vi "Generate Comments.vi"(7 "error in (no error)":errorcluster, 9 "cluster":T1) -> (0 "error out":errorcluster, 3 "Comments":string)   [LabVIEW 2016, in "Control Experiment.lvclass"]
uses:
  Control Experiment.lvclass
  Typedefs/Comments-cluster.ctl
  <userlib>/LevyLab/Krohn Hite 7008/typedefs/Gain-Enum.ctl
  <userlib>/LevyLab/Krohn Hite 7008/typedefs/Input Configuration-Enum.ctl
  <userlib>/LevyLab/Krohn Hite 7008/typedefs/Shunt-Enum.ctl
  <userlib>/LevyLab/Krohn Hite 7008/KH7008.lvclass
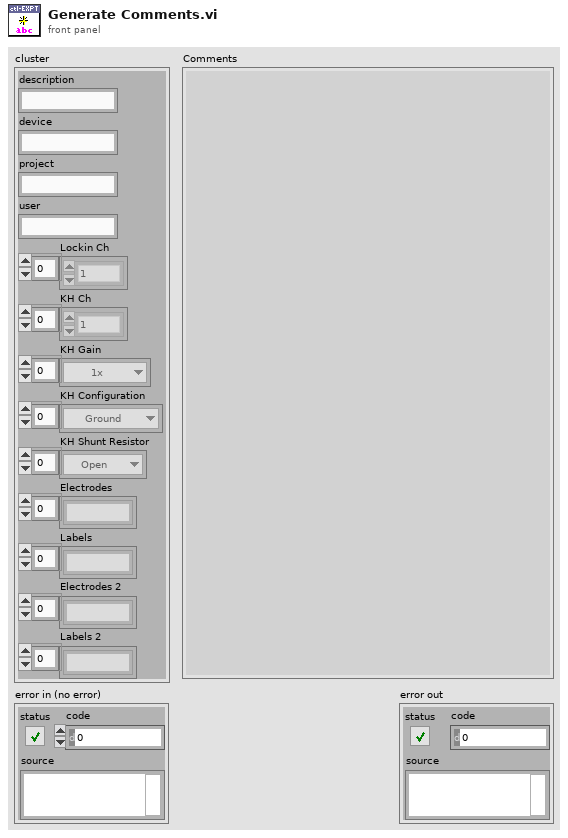
[diagram p1: front panel]
types:
  T1 = typedef "Control Experiment.lvclass/Comments-cluster.ctl" = cluster{"description":string, "device":string, "project":string, "user":string, "Lockin Ch":enum16{"1", "2", "3", "4", "5", "6", "7", "8"}[], "KH Ch":enum16{"1", "2", "3", "4", "5", "6", "7", "8"}[], "KH Gain":T2[], "KH Configuration":T3[], "KH Shunt Resistor":T4[], "Electrodes":string[], "Labels":string[], "Electrodes 2":string[], "Labels 2":string[]}
  T2 = typedef "KH7008.lvclass/Gain-Enum.ctl" = enum16{"1x", "10x", "100x", "1000x"}
  T3 = typedef "KH7008.lvclass/Input Configuration-Enum.ctl" = enum16{"Ground", "SE+ (-gnd)", "SE- (+gnd)", "Differential"}
  T4 = typedef "KH7008.lvclass/Shunt-Enum.ctl" = enum16{"Open", "50 Ohms", "500 Ohms", "5k Ohms", "50k Ohms"}
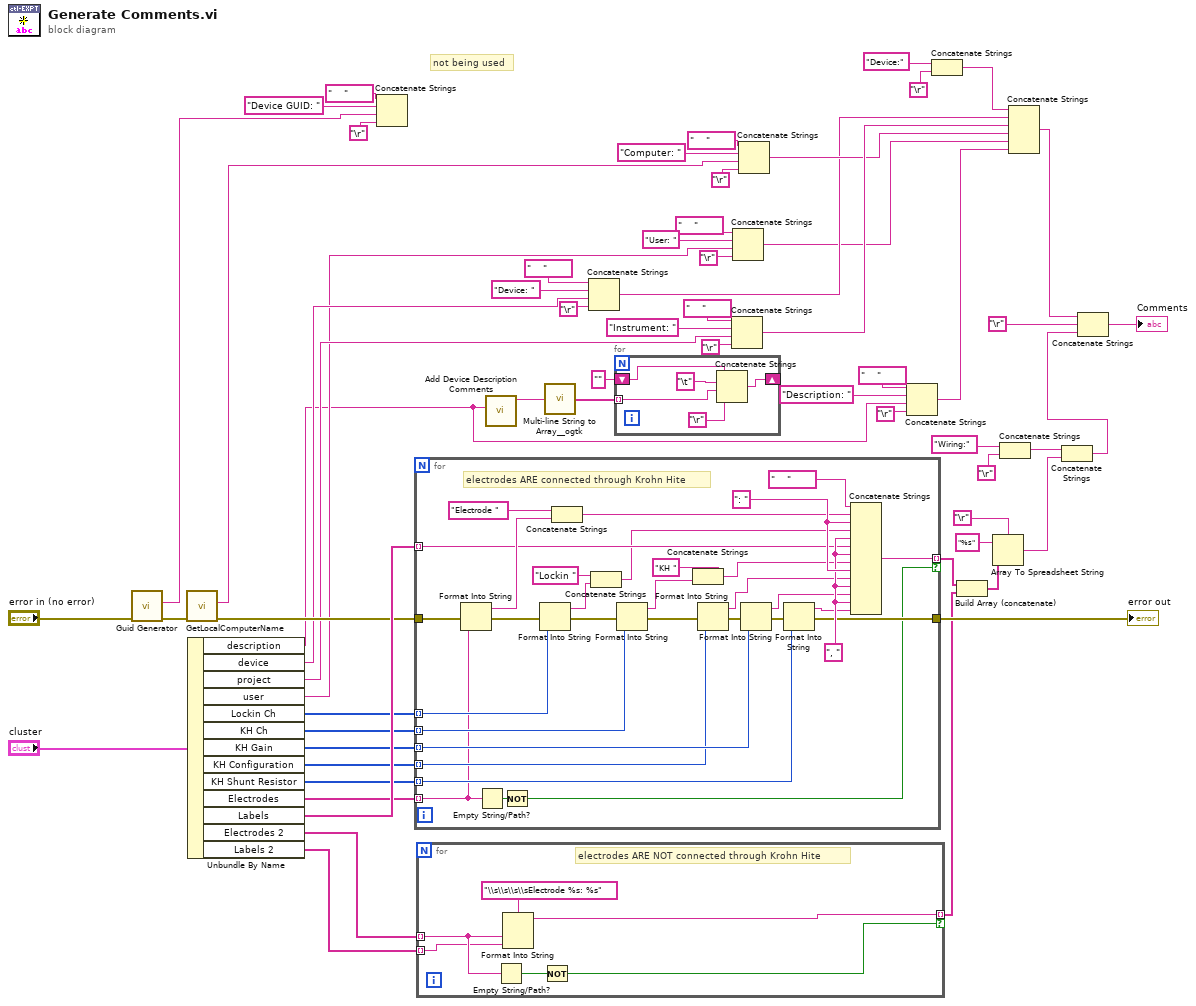
[diagram p0: block diagram]
diagram:
  # "not being used"
  n1 = call <vilib>:"Guid Generator.vi"("error in (no error)"="error in (no error)") -> ("error out"=w41:errorcluster, "GUID"=w29:string)  [unwired: 9 in]
  n2 = call <userlib>:"GetLocalComputerName.vi"("error in (no error)"=w41) -> ("error out"=w52:errorcluster, "Name"=w25:string)  [unwired: 9 in]
  n3 = Unbundle By Name("cluster") -> ("description"=w5:string, "device"=w45:string, "project"=w44:string, "user"=w43:string, "Lockin Ch"=w56:enum16{"1", "2", "3", "4", "5", "6", "7", "8"}[], "KH Ch"=w57:enum16{"1", "2", "3", "4", "5", "6", "7", "8"}[], "KH Gain"=w58:T2[], "KH Configuration"=w59:T3[], "KH Shunt Resistor"=w60:T4[], "Electrodes"=w61:string[], "Labels"=w62:string[], "Electrodes 2"=w14:string[], "Labels 2"=w15:string[])
  n4 = Concatenate Strings("    " ("string"), "Device GUID: " ("string"), w29, "\r") -> ()  [unwired: 1 out]
  n5 = for {
    tunnel: w56 -> [w76] mode=indexing
    tunnel: w57 -> [w77] mode=indexing
    tunnel: w58 -> [w79] mode=indexing
    tunnel: w59 -> [w78] mode=indexing
    tunnel: w60 -> [w80] mode=indexing
    tunnel: w61 -> [w67] mode=indexing
    tunnel: w62 -> [w81] mode=indexing
    tunnel: [w91] -> w2 mode=indexing if=w65
    tunnel: w52 -> [w74]
    tunnel: [w82] -> w51
    w88 = ", "
    w89 = ": "
    # "electrodes ARE connected through Krohn Hite"
    n6 = Format Into String(error in=w74, w67) -> (resulting string=w90:string, error out=w73:errorcluster)  [unwired: 2 in]
    n7 = Empty String/Path?(string/path=w67) -> (empty?=w66:bool)
    n8 = Not(x=w66) -> (.not. x?=w65:bool)
    n9 = Format Into String(error in=w73, w76) -> (resulting string=w93:string, error out=w72:errorcluster)  [unwired: 2 in]
    n10 = Concatenate Strings("Electrode ", w90) -> (w64:string)
    n11 = Concatenate Strings("Lockin ", w93) -> (w63:string)
    n12 = Format Into String(error in=w72, w77) -> (resulting string=w71:string, error out=w85:errorcluster)  [unwired: 2 in]
    n13 = Concatenate Strings("KH ", w71) -> (w70:string)
    n14 = Format Into String(error in=w85, w78) -> (resulting string=w69:string, error out=w84:errorcluster)  [unwired: 2 in]
    n15 = Format Into String(error in=w84, w79) -> (resulting string=w68:string, error out=w83:errorcluster)  [unwired: 2 in]
    n16 = Format Into String(error in=w83, w80) -> (resulting string=w87:string, error out=w82:errorcluster)  [unwired: 2 in]
    n17 = Concatenate Strings("    " ("string"), w64, w89, w63, w88, w81, w88, w70, w89, w69, w88, w68, w88, w87) -> (w91:string)
  }
  "error out" <- w51
  n18 = for {
    tunnel: [w95] -> w3 mode=indexing if=w97
    tunnel: w15 -> [w96] mode=indexing
    tunnel: w14 -> [w99] mode=indexing
    # "electrodes ARE NOT connected through Krohn Hite"
    n19 = Empty String/Path?(string/path=w99) -> (empty?=w98:bool)
    n20 = Format Into String(format string="\\s\\s\\s\\sElectrode %s: %s", w99, w96) -> (resulting string=w95:string)  [unwired: 2 in, 1 out]
    n21 = Not(x=w98) -> (.not. x?=w97:bool)
  }
  n22 = call "Add Device Description Comments.vi"("Device Description"=w5) -> ("Comments"=w17:string)  [unwired: 8 in, 1 out]
  n23 = call <userlib>:"Multi-line String to Array__ogtk.vi"("string"=w17) -> ("lines"=w16:string[])
  n24 = Concatenate Strings("    " ("string"), "Device: " ("string"), w45, "\r") -> (w11:string)
  n25 = for {
    tunnel: w16 -> [w102] mode=indexing
    shift-right: [w105] -> _
    shift-left: "" ("string") -> [w103]
    n26 = Concatenate Strings(w103, "\t" ("string"), w102, "\r") -> (w105:string)
  }
  n27 = Concatenate Strings("    " ("string"), "Instrument: " ("string"), w44, "\r") -> (w13:string)
  n28 = Concatenate Strings("    " ("string"), "User: " ("string"), w43, "\r") -> (w10:string)
  n29 = Concatenate Strings("    " ("string"), "Computer: " ("string"), w25, "\r") -> (w12:string)
  n30 = Concatenate Strings("    " ("string"), "Description: " ("string"), w5, "\r") -> (w7:string)
  n31 = Concatenate Strings("Device:" ("string"), "\r") -> (w33:string)
  n32 = Build Array (concatenate)(w2, w3) -> (w1:string[])
  n33 = Array To Spreadsheet String(delimiter (Tab)="\r", array=w1, 3:"%s" ("format string")) -> (spreadsheet string=w20:string)
  n34 = Concatenate Strings("Wiring:" ("string"), "\r") -> (w21:string)
  n35 = Concatenate Strings(w33, w11, w13, w12, w10, w7) -> (w24:string)
  n36 = Concatenate Strings(w21, w20) -> (w19:string)
  n37 = Concatenate Strings(w24, "\r", w19) -> (→"Comments":string)
